vi "CheckValueChange.vi"(1 "Button Down":bool) -> (0 "Boolean":bool)   [LabVIEW 2015]
doc: "Checks for a value change"
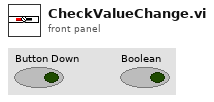
[diagram p1: front panel]
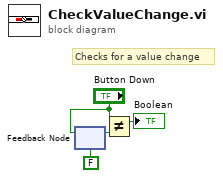
[diagram p0: block diagram]
diagram:
  # "Checks for a value change"
  n1 = feedback #1(FALSE ("Button Down")) -> (w2:bool)
  n2 = feedback-in #1("Button Down") -> ()
  n3 = Not Equal?(x="Button Down", y=w2) -> (x != y?=→"Boolean":bool)
